vi "MultiAxisMove.vi"(5 "Find Location":bool, 6 "error in":errorcluster, 7 "Wait For Move Complete":bool, 8 "Position Mode (Rel)":T1(ring)=enum."Relative Position", 9 "Distance to move (mm)":dbl[](array[numeric]), 10 "Move Polarity":i32=1, 11 "Motion Settings":T2={"No Motion?"=FALSE, "Motion System"=enum."MM3000", "Motion Bd ID"=0, "Motion Profile"="SMAC1", "# Axis"=0, "Reverse Z axis?"=FALSE, "SMAC Axis"=0, "scan pair"=enum."y-(x) scan", "RT fps"=0.0, "Steps per mm"=[], "Motor Parameters"={"velocity ct/s"=[], "accel ct/s^2"=[]}, "One Way Scan"=FALSE, "Reverse One Way Scan"=FALSE, "Global Position (mm)"=[], "Plane"=0, "Distance between\nscan lines (um)"=0.0, "Distance between\nscan planes (um)"=0.0, "number of scan planes"=0, "Total steps in line"=0, "Xtra plane\ndistance  (um)"=0, "Xtra planes "=0, "Add Axis"=FALSE, "overshoot cts"=0, "BKPT Shift"=0, "Scan Start Time (ms)"=0, "ESP VISA"="", "3rd Axis"=1, "GL Ref Out"=refnum, "Galil Address"=""} {"3rd Axis" items=["x", "y", "z", "w"]; "Xtra planes" min=1; "Xtra plane\ndistance  (um)" min=0; "Distance between\nscan planes (um)" format="%.2f"; "Distance between\nscan lines (um)" format="%.2f"; "SMAC Axis" items=["None"=0, "Axis 1"=1, "Axis 2"=2, "Axis 3"=3, "Axis 4"=4, "Axis 5"=5, "Axis 6"=6, "Axis 7"=7, "Axis 8"=8, "Vector Space 1"=17, "Vector Space 2"=18, "Vector Space 3"=19, "Vector Space 4"=20]; "Motion Bd ID" min=1 max=32 step=1}) -> (0 "error out":errorcluster, 1 "location (mm)":dbl[](array[numeric]), 3 "Motion Settings Out":T2={"No Motion?"=FALSE, "Motion System"=enum."NI 735x", "Motion Bd ID"=1, "Motion Profile"="SMAC1", "# Axis"=1, "Reverse Z axis?"=TRUE, "SMAC Axis"=0, "scan pair"=enum."y-(x) scan", "RT fps"=6.0, "Steps per mm"=[1000, 1000, 1000, 1000], "Motor Parameters"={"velocity ct/s"=[10000.0, 10000.0, 10000.0, 50000.0], "accel ct/s^2"=[50000.0, 50000.0, 50000.0, 200000.0]}, "One Way Scan"=FALSE, "Reverse One Way Scan"=FALSE, "Global Position (mm)"=[], "Plane"=0, "Distance between\nscan lines (um)"=0.0, "Distance between\nscan planes (um)"=0.0, "number of scan planes"=1, "Total steps in line"=0, "Xtra plane\ndistance  (um)"=100, "Xtra planes "=1, "Add Axis"=FALSE, "overshoot cts"=200, "BKPT Shift"=0, "Scan Start Time (ms)"=0, "ESP VISA"="GPIB::1::INSTR", "3rd Axis"=1, "GL Ref Out"=refnum, "Galil Address"=""} {"3rd Axis" items=["x", "y", "z", "w"]; "Xtra planes" min=1; "Xtra plane\ndistance  (um)" min=0; "Distance between\nscan planes (um)" format="%.2f"; "Distance between\nscan lines (um)" format="%.2f"; "SMAC Axis" items=["None"=0, "Axis 1"=1, "Axis 2"=2, "Axis 3"=3, "Axis 4"=4, "Axis 5"=5, "Axis 6"=6, "Axis 7"=7, "Axis 8"=8, "Vector Space 1"=17, "Vector Space 2"=18, "Vector Space 3"=19, "Vector Space 4"=20]; "Motion Bd ID" min=1 max=32 step=1})   [LabVIEW 2022 SP3]
uses:
  NI_controller/-NI_MotionRoutines/MotionParameters.ctl
  NI_controller/-NI_MotionRoutines/MotionSys.ctl
  ScanAxis.ctl
  3rdAxis.ctl
  Galil/Command Menu.ctl
  MotionGlobals.vi
  <vilib>/Motion/FlexMotion/FunctionsVIs/StartStopMotion.llb/Start Motion (8 axes).flx
panel:
  # "1-D and 2-D B scan settings"
  # "1-D and 2-D B scan settings"
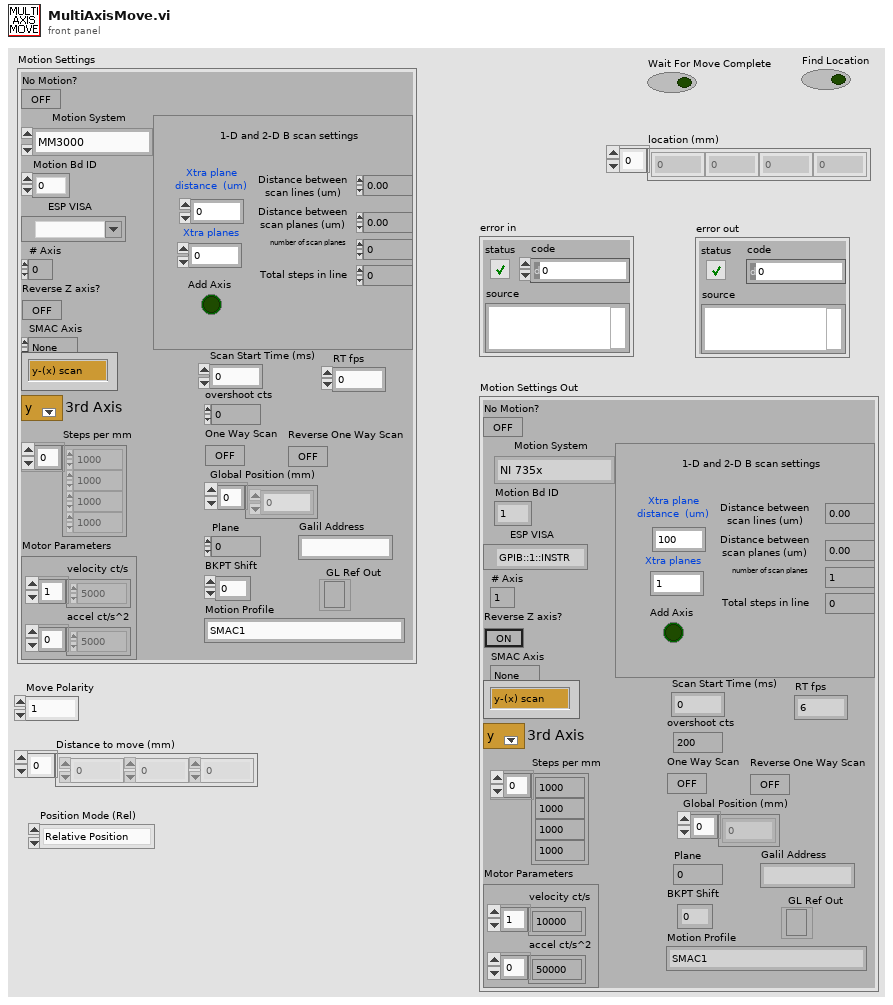
[diagram p1: front panel]
types:
  T1 = enum16{"Absolute Position", "Relative Position", "Velocity", "Relative to Cap Pos", "Modulus Position", "Absolute Contouring", "Relative Contouring"}
  T2 = typedef "MotionParameters.ctl" = cluster{"No Motion?":bool, "Motion System":T3, "Motion Bd ID":u8, "Motion Profile":string, "# Axis":i8, "Reverse Z axis?":bool, "SMAC Axis":u16, "scan pair":T4, "RT fps":sgl, "Steps per mm":i32[], "Motor Parameters":cluster{"velocity ct/s":dbl[], "accel ct/s^2":dbl[]}, "One Way Scan":bool, "Reverse One Way Scan":bool, "Global Position (mm)":dbl[], "Plane":i32, "Distance between\nscan lines (um)":sgl, "Distance between\nscan planes (um)":sgl, "number of scan planes":i32, "Total steps in line":i32, "Xtra plane\ndistance  (um)":i32, "Xtra planes ":i32, "Add Axis":bool, "overshoot cts":i32, "BKPT Shift":i32, "Scan Start Time (ms)":u32, "ESP VISA":refnum<visa-resource-name>, "3rd Axis":T5, "GL Ref Out":refnum<k7>, "Galil Address":string}
  T3 = typedef "MotionSys.ctl" = enum16{"MM3000", "NI 735x", "Newport ESP", "No Motion Card", "Galil"}
  T4 = typedef "ScanAxis.ctl" = enum16{"y-(x) scan", "x-(y) scan", "z-(x) scan", "z-(y) scan", "y-(z) scan", "x-(z) scan", "w-(x) scan", "w-(y) scan", "w-(z) scan", "x-(w) scan", "y-(w) scan", "z-(w) scan"}
  T5 = typedef "3rdAxis.ctl" = u16
  T6 = typedef "location.ctl" = enum16{"Automatic", "WCM Main", "Hawaii", "Columbia MM3000", "Columbia  NI System", "NYU", "RRI 2", "UHI Allen", "CUMC RT", "Chiba", "Stony Brook", "WCM Microscopy", "WCM Aeoretch", "WCM Optics Lab", "WCM Main 2Axis", "WCM Rotation", "WCM SAM SMAC", "SERI GP"}
  T7 = typedef "Command Menu.ctl" = enum16{"CommandPassThrough", "Abort Motion", "Define Pos", "Velocity", "Acceleration", "Deceleration", "Position Rel", "Postion Abs", "Begin Move", "After Move", "Home", "KI", "KD", "KP", "IL", "Config I/O", "Set Bit", "Clear Bit", "Motor Off", "Moto On", "Status", "Execute", "Halt Execute", "HX Status", "Tell Velocity", "Check Motion", "BreakPoint", "Tell Position", "Current Code Line", "Tell Switches", "OC Force On", "OC Off", "Pos Soft Limit", "Rev Soft Limit"}
  T8 = typedef "Resource Out (Enum).flx" = u16
  T9 = typedef "Bd Id Out" = u8
  T10 = typedef "GL Axis Control.ctl" = u16
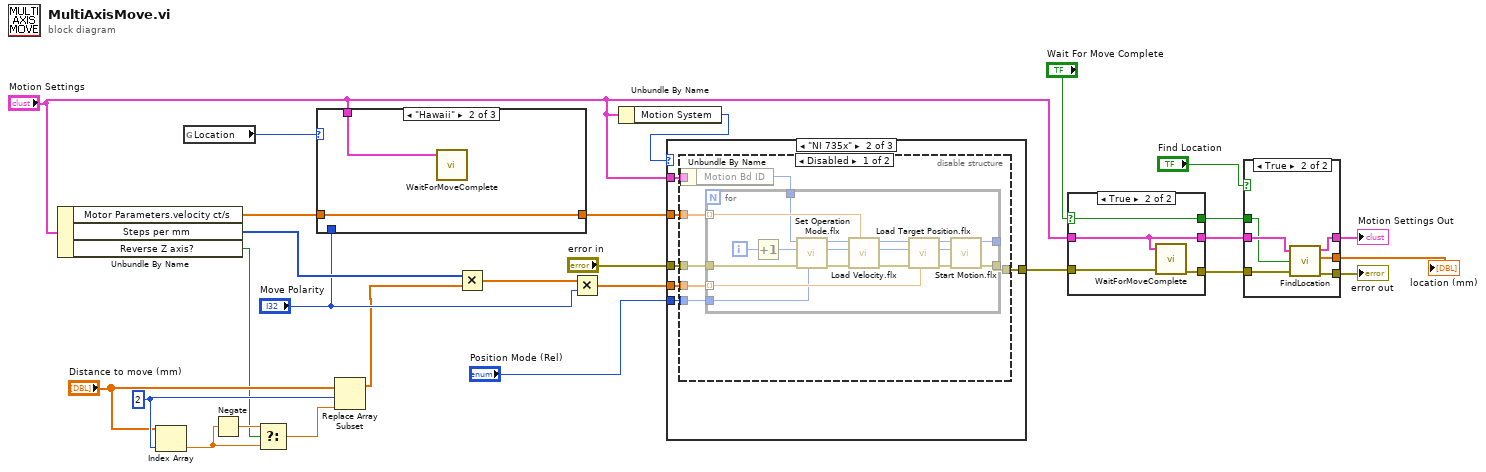
[diagram p0: block diagram]
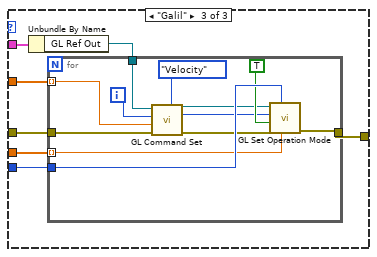
[diagram p4: hidden frame]
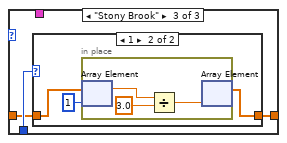
[diagram p6: hidden frame]
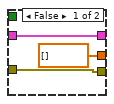
[diagram p8: hidden frame]
diagram:
  w6 = 2 ("index")
  n1 = Unbundle By Name("Motion Settings") -> ("Motor Parameters.velocity ct/s"=w11:dbl[], "Steps per mm"=w14:i32[], "Reverse Z axis?"=w1:bool)
  n2 = Index Array(array="Distance to move (mm)", index=w6) -> (element=w8:dbl)
  n3 = global read "MotionGlobals.vi" "Location"() -> (w13:T6)
  n4 = Negate(x=w8) -> (-x=w9:dbl)
  n5 = Select(t=w9, s=w1, f=w8) -> (s? t:f=w7:dbl)
  n6 = case shown="\"Hawaii\"" w13 {
    tunnel: [w28 w30 w31] -> w12
    tunnel: w11 -> [w28 w30 w32]
    tunnel: "Move Polarity" -> [_ _ w33]
    tunnel: "Motion Settings" -> [_ w29 _]
    frame "WCM Main", Default {
    }
    frame "Hawaii" {
      n7 = call "WaitForMoveComplete.vi"("Motion Settings"=w29) -> ()  [unwired: 5 in, 1 out]
    }
    frame "Stony Brook" {
      n8 = case shown="1" w33 {
        tunnel: [w34 w36] -> w31
        tunnel: w32 -> [w34 w37]
        frame 0, Default {
        }
        frame 1 {
          n9 = in-place {
            n10 = in-place-array #1(w37, 1) -> (w39:dbl)
            n11 = Divide(x=w39, y=3.0) -> (x/y=w40:dbl)
            n12 = in-place-array #1(w40) -> (w36:dbl[])  [unwired: 1 out]
          }
        }
      }
    }
  }
  n13 = Replace Array Subset(array="Distance to move (mm)", new element=w7, index=w6) -> (w4:dbl[])
  n14 = Multiply(x=w14, y=w4) -> (x*y=w27:dbl[])
  n15 = Multiply(x=w27, y="Move Polarity") -> (x*y=w25:dbl[])
  n16 = Unbundle By Name("Motion Settings") -> ("Motion System"=w2:T3)
  n17 = case shown="\"NI 735x\"" w2 {
    tunnel: "error in" -> [w41 w47 w78]
    tunnel: w25 -> [_ w46 w77]
    tunnel: "Position Mode (Rel)" -> [_ w45 w76]
    tunnel: [w41 w44 w75] -> w22
    tunnel: w12 -> [_ w43 w74]
    tunnel: "Motion Settings" -> [_ w42 w73]
    frame "MM3000", Default {
    }
    frame "NI 735x" {
      n18 = disable-structure shown="Disabled" {
        disable-tunnel: w47 -> [w54 _]
        disable-tunnel: w46 -> [w53 _]
        disable-tunnel: w45 -> [w52 _]
        disable-tunnel: [w51 _] -> w44
        disable-tunnel: w43 -> [w50 _]
        disable-tunnel: w42 -> [w49 _]
        frame Disabled {
          n19 = Unbundle By Name(w49) -> ("Motion Bd ID"=w48:u8)
          n20 = for {
            tunnel: w53 -> [w65] mode=indexing
            tunnel: [w68] -> w51
            tunnel: [w67] -> _
            tunnel: w54 -> [w66]
            tunnel: w52 -> [w63]
            tunnel: w50 -> [w58] mode=indexing
            tunnel: w48 -> [w55]
            i -> [w64]
            n21 = Increment(x=w64) -> (x+1=w62:i32)
            n22 = call <vilib>:"Set Operation Mode.flx"("Position Mode (Absolute)"=w63, "error in (no error)"=w66, "Axis or Vector Space"=w62, "Board ID"=w55) -> ("error out"=w61:errorcluster, "Resource Output"=w56:T8, "Bd ID Out"=w57:T9)  [unwired: 2 out]
            n23 = call <vilib>:"Load Velocity.flx"("Velocity (10000)"=w58, "error in (no error)"=w61, "Axis or Vector Space"=w56, "Board ID"=w57) -> ("Resource Output"=w59:T8, "Bd ID Out"=w60:T9)  [unwired: 3 in, 1 out]
            n24 = call <vilib>:"Load Target Position.flx"("Target Position (0)"=w65, "error in (no error)"=w61, "Axis"=w59, "Board ID"=w60) -> ("error out"=w70:errorcluster, "Resource Output"=w69:T8, "Bd ID Out"=w71:T9)  [unwired: 3 out]
            n25 = call-poly <vilib>:"Start Motion.flx"("error in (no error)"=w70, "Axis or Vector Space"=w69, "Board ID"=w71) -> ("error out"=w68:errorcluster, "Bd ID Out"=w67:T9)  [unwired: 1 in, 3 out]
          }
        }
        frame Enabled {
        }
      }
    }
    frame "Galil" {
      n26 = Unbundle By Name(w73) -> ("GL Ref Out"=w72:refnum<k7>)
      n27 = for {
        tunnel: w77 -> [w89] mode=indexing
        tunnel: [w79] -> w75
        tunnel: w78 -> [w81]
        tunnel: w76 -> [w90]
        tunnel: w74 -> [w84] mode=indexing
        tunnel: w72 -> [w87]
        i -> [w83]
        n28 = call "GL Command Set.vi"("Command"=Command_Menu."Velocity", "error in (no error)"=w81, "Value"=w84, "Axis"=w83, "Galil.IGalil"=w87) -> ("error out"=w80:errorcluster, "Axis Out"=w82:T10, "ref out"=w85:refnum<k7>)  [unwired: 2 in, 2 out]
        n29 = call "GL Set Operation Mode.vi"("position cts (abs/rel)"=w89, "Position Mode (Absolute)"=w90, "error in (no error)"=w80, "Start Now?"=TRUE, "Axis"=w82, "Galil.IGalil"=w85) -> ("error out"=w79:errorcluster)  [unwired: 3 in, 2 out]
      }
    }
  }
  n30 = case shown="True" "Wait For Move Complete" {
    selector: "Wait For Move Complete" -> [w91 w94]
    tunnel: [w93 w97] -> w21
    tunnel: w22 -> [w93 w96]
    tunnel: "Motion Settings" -> [w92 w95]
    tunnel: [w92 w95] -> w18
    tunnel: [w91 w94] -> w15
    frame False {
    }
    frame True {
      n31 = call "WaitForMoveComplete.vi"("Motion Settings"=w95, "error in"=w96) -> ("error out"=w97:errorcluster)  [unwired: 4 in]
    }
  }
  n32 = case shown="True" "Find Location" {
    tunnel: w21 -> [w99 w106]
    tunnel: [w99 w105] -> w20
    tunnel: [w100 w104] -> w19
    tunnel: w18 -> [w100 w103]
    tunnel: [dbl[] [] ("location (mm)") w102] -> w16
    tunnel: w15 -> [_ w101]
    frame False {
    }
    frame True {
      n33 = call "FindLocation.vi"("Motion Settings"=w103, "Wait for Motion Complete"=w101, "error in (no error)"=w106) -> ("Motion Settings Out"=w104:T2, "location (mm)"=w102:dbl[], "error out"=w105:errorcluster)  [unwired: 1 out]
    }
  }
  "error out" <- w20
  "Motion Settings Out" <- w19
  "location (mm)" <- w16
